vi "GetParam.vi"(8 "error in (no error)":errorcluster caption="entrée d'erreur (pas d'erreur)", 11 "Normalizer.lvclass":refnum<class "Normalizer.lvclass">) -> (0 "error out":errorcluster caption="sortie d'erreur", 2 "Normalizer":cluster{"norm":string, "copy":bool}={"norm"="l2", "copy"=TRUE}, 3 "Normalizer.lvclass":refnum<class "Normalizer.lvclass">)   [LabVIEW 2020, in "Normalizer.lvclass"]
doc: "Get Parameters"
uses:
  Normalizer.lvclass
  Normalizer.lvclass/Normalizer.ctl
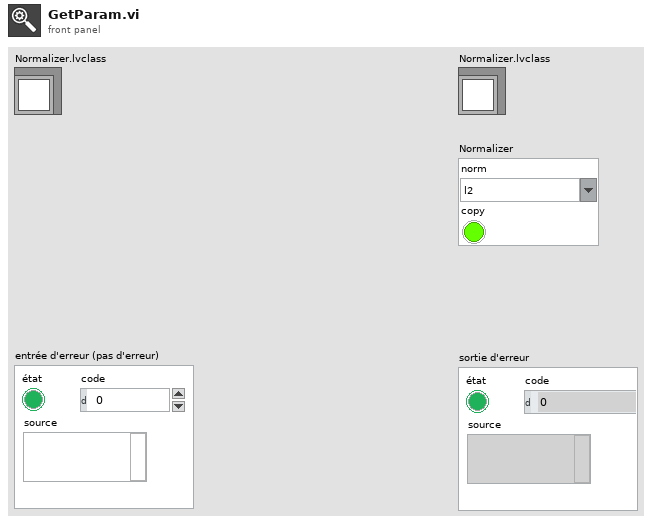
[diagram p1: front panel]
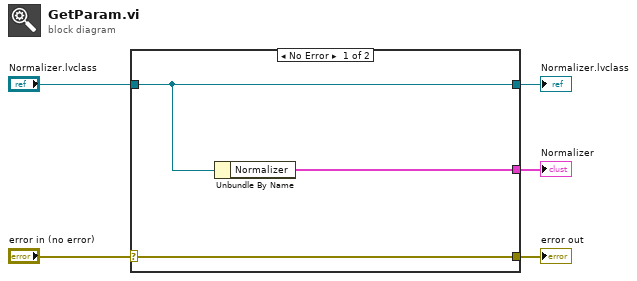
[diagram p0: block diagram]
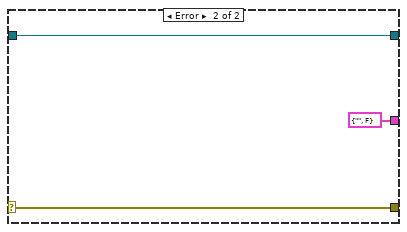
[diagram p2: hidden frame]
diagram:
  n1 = case shown="No Error" "error in (no error)" {
    selector: "error in (no error)" -> [w8 w10]
    tunnel: [w8 w10] -> w4
    tunnel: [w7 w11] -> w2
    tunnel: "Normalizer.lvclass" -> [w7 w11]
    tunnel: [w6 cluster{"norm":string, "copy":bool} {"norm"="", "copy"=FALSE} ("Normalizer")] -> w1
    frame No Error {
      n2 = Unbundle By Name(w7) -> ("Normalizer"=w6:cluster{"norm":string, "copy":bool})
    }
    frame Error {
    }
  }
  "error out" <- w4
  "Normalizer.lvclass" <- w2
  "Normalizer" <- w1
